vi "test_struct_abs_conventional.vi"() -> ()   [LabVIEW 2017]
doc: "Minimal example that demonstrates functions implemented in the SorpPropLib for absorption working pairs based on the conventional approach."
panel:
  out "Der. of concentration wrt. pressure":cluster{dbl[], dbl[]}[](graph)
  out "Der. of concentration wrt. temperature":cluster{dbl[], dbl[]}[](graph)
  out "Der. of pressure wrt. concentration":cluster{dbl[], dbl[]}[](graph)
  out "Der. of pressure wrt. temperature":cluster{dbl[], dbl[]}[](graph)
  out "Temperature":cluster{dbl[], dbl[]}[](graph)
  out "Pressure":cluster{dbl[], dbl[]}[](graph)
  out "Concentration":cluster{dbl[], dbl[]}[](graph)
  in  "WorkingPair (Input)":T1={"no_iso"=1, "no_p_sat"=1, "path_db"="D:\\Driesel\\SorpLibLocal\\labview_wrapper\\data\\json\\sorpproplib.json", "wp_as"="NaOH-KOH-CsOH", "wp_st"="", "wp_iso"="Duehring", "wp_rf"="Water", "rf_rhol"="SaturatedLiquidDensity_EoS1", "no_rhol"=1, "rf_psat"="VaporPressure_EoS1"}
  in  "Temperature in K (Input)":dbl=353.0
  in  "Pressure in Pa (Input)":dbl=1000.0
  # "Increase pressure by 5000 Pa in steps of 1 Pa."
  # "Path to database"
  # "Name of sorbent"
  # "Name of sub-type of sorbent"
  # "Name of refrigerant"
  # "Name of isotherm"
  # "ID of isotherm"
  # "Name of calculation approach for vapor pressure"
  # "ID of vapor pressure equation"
  # "Name of calculation approach for liquid density"
  # "ID of liquid density equation"
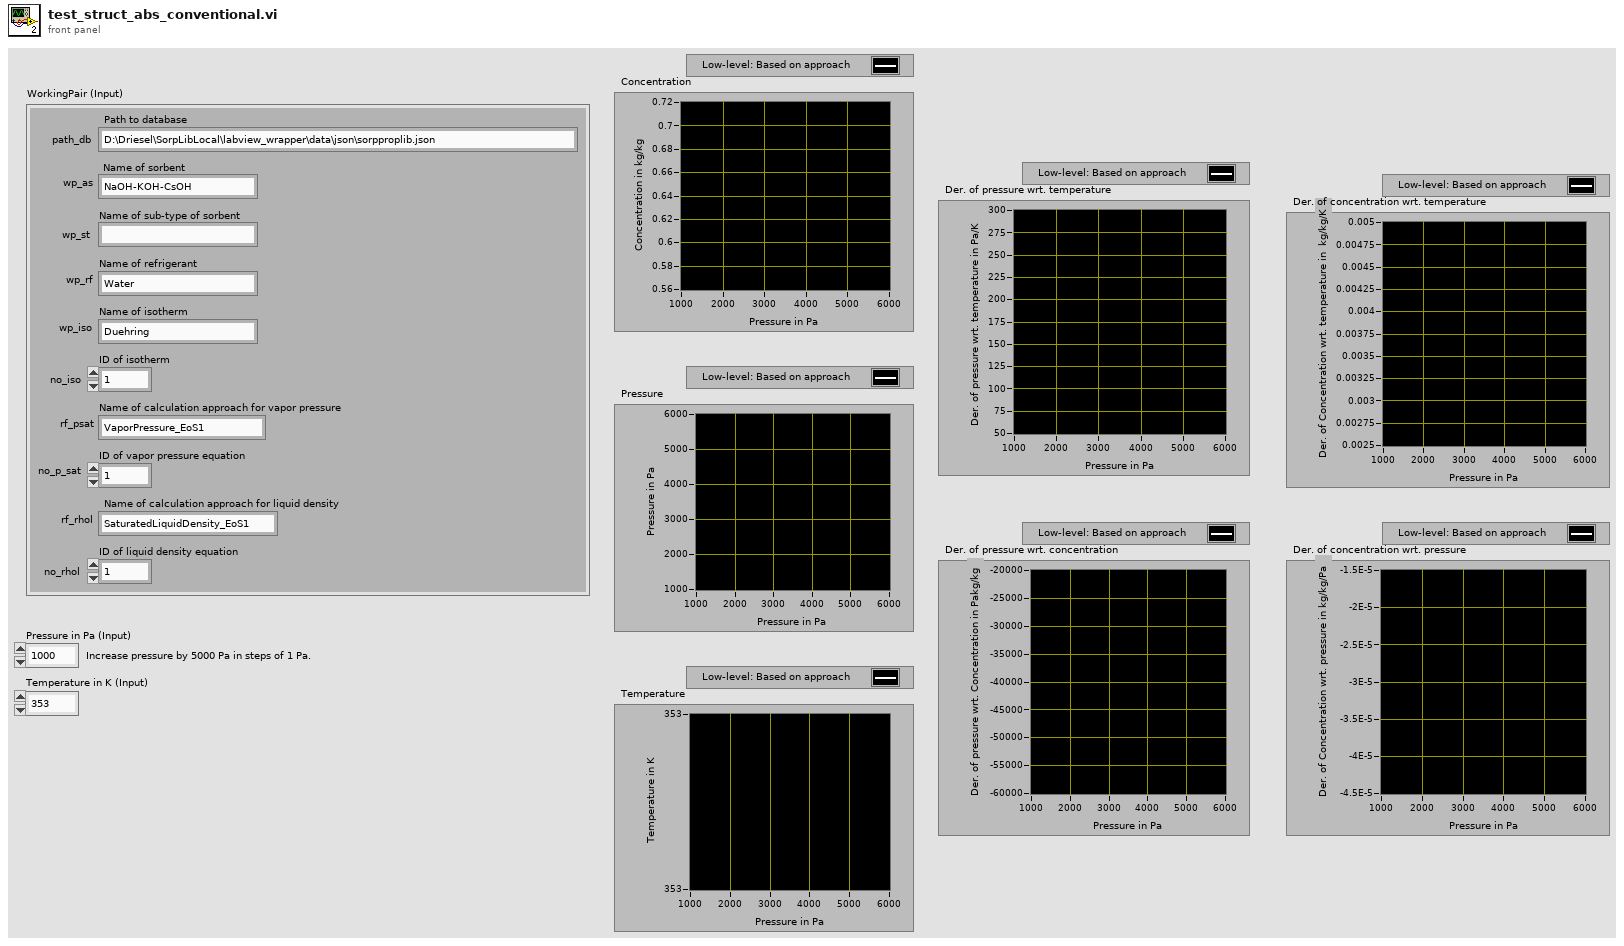
[diagram p1: front panel]
types:
  T1 = cluster{"no_iso":i32, "no_p_sat":i32, "path_db":string, "wp_as":string, "wp_st":string, "wp_iso":string, "wp_rf":string, "rf_rhol":string, "no_rhol":i32, "rf_psat":string}
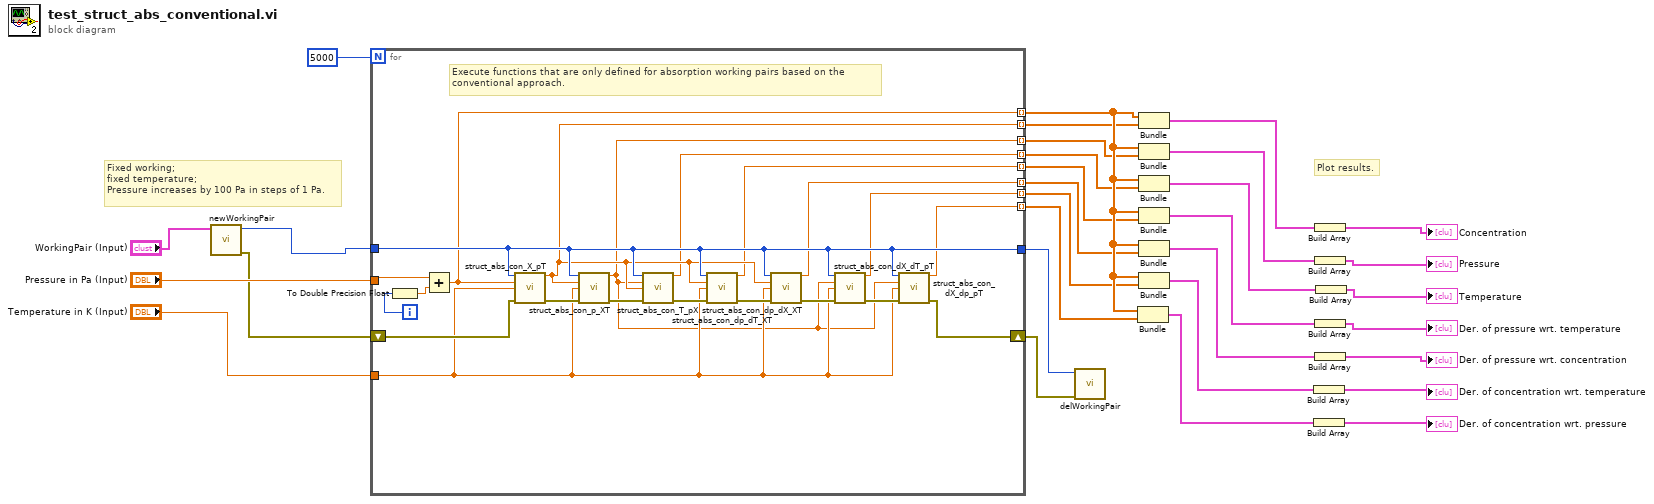
[diagram p0: block diagram]
diagram:
  # "Plot results."
  # "Fixed working;\nfixed temperature;\nPressure increases by 100 Pa in steps of 1 Pa."
  n1 = call "newWorkingPair.vi"("WorkingPair (Input)"="WorkingPair (Input)") -> ("Error (Output)"=w17:errorcluster, "workingPair"=w18:i64)  [unwired: 9 in]
  n2 = for {
    N: 5000 -> [_]
    tunnel: "Pressure in Pa (Input)" -> [w51]
    tunnel: "Temperature in K (Input)" -> [w38]
    tunnel: w18 -> [w40]
    shift-right: [w41] -> w16
    shift-left: w17 -> [w48]
    tunnel: [w39] -> w28 mode=indexing
    tunnel: [w40] -> w15
    tunnel: [w37] -> w14 mode=indexing
    tunnel: [w36] -> w13 mode=indexing
    tunnel: [w35] -> w12 mode=indexing
    tunnel: [w34] -> w11 mode=indexing
    tunnel: [w33] -> w10 mode=indexing
    tunnel: [w32] -> w9 mode=indexing
    tunnel: [w31] -> w8 mode=indexing
    i -> [w50]
    # "Execute functions that are only defined for absorption working pairs based on the\nconventional approach."
    n3 = To Double Precision Float(number=w50) -> (double precision float=w49:dbl)
    n4 = Add(x=w51, y=w49) -> (x+y=w39:dbl)
    n5 = call "struct_abs_con_X_pT.vi"("Reference working pair (Input)"=w40, "Pressure in Pa (Input)"=w39, "Temperature in K (Input)"=w38, "Error (Input)"=w48) -> ("Concentration in kg/kg (Output)"=w37:dbl, "Error (Output)"=w47:errorcluster)  [unwired: 10 in]
    n6 = call "struct_abs_con_p_XT.vi"("Reference working pair (Input)"=w40, "Concentration in kg/kg (Input)"=w37, "Temperature in K (Input)"=w38, "Error (Input)"=w47) -> ("Pressure in Pa (Output)"=w36:dbl, "Error (Output)"=w46:errorcluster)  [unwired: 10 in]
    n7 = call "struct_abs_con_T_pX.vi"("Reference working pair (Input)"=w40, "Pressure in Pa (Input)"=w36, "Concentration in kg/kg (Input)"=w37, "Error (Input)"=w46) -> ("Temperature in K (Output)"=w35:dbl, "Error (Output)"=w45:errorcluster)  [unwired: 10 in]
    n8 = call "struct_abs_con_dp_dT_XT.vi"("Reference working pair (Input)"=w40, "Concentration in kg/kg (Input)"=w37, "Temperature in K (Input)"=w38, "Error (Input)"=w45) -> ("Der. of equilibrium pressure wrt. temperature in Pa/K (Output)"=w34:dbl, "Error (Output)"=w44:errorcluster)  [unwired: 10 in]
    n9 = call "struct_abs_con_dp_dX_XT.vi"("Reference working pair (Input)"=w40, "Concentration in kg/kg (Input)"=w37, "Temperature in K (Input)"=w38, "Error (Input)"=w44) -> ("Der. of equilibrium pressure wrt. concentration in Pakg/kg (Output)"=w33:dbl, "Error (Output)"=w43:errorcluster)  [unwired: 10 in]
    n10 = call "struct_abs_con_dX_dT_pT.vi"("Reference working pair (Input)"=w40, "Pressure in Pa (Input)"=w36, "Temperature in K (Input)"=w38, "Error (Input)"=w43) -> ("Der. of equilibrium concentration wrt. temperature in kg/kg/K (Output)"=w32:dbl, "Error (Output)"=w42:errorcluster)  [unwired: 10 in]
    n11 = call "struct_abs_con_dX_dp_pT.vi"("Reference working pair (Input)"=w40, "Pressure in Pa (Input)"=w36, "Temperature in K (Input)"=w38, "Error (Input)"=w42) -> ("Der. of equilibrium concentration wrt. pressure in kg/kg/Pa (Output)"=w31:dbl, "Error (Output)"=w41:errorcluster)  [unwired: 10 in]
  }
  n12 = call "delWorkingPair.vi"("Error (Input)"=w16, "workingPair"=w15) -> ()  [unwired: 9 in, 1 out]
  n13 = Bundle(w28, w8) -> (w21:cluster{dbl[], dbl[]})  [unwired: 1 in]
  n14 = Bundle(w28, w14) -> (w27:cluster{dbl[], dbl[]})  [unwired: 1 in]
  n15 = Bundle(w28, w13) -> (w26:cluster{dbl[], dbl[]})  [unwired: 1 in]
  n16 = Bundle(w28, w12) -> (w25:cluster{dbl[], dbl[]})  [unwired: 1 in]
  n17 = Bundle(w28, w11) -> (w24:cluster{dbl[], dbl[]})  [unwired: 1 in]
  n18 = Bundle(w28, w10) -> (w23:cluster{dbl[], dbl[]})  [unwired: 1 in]
  n19 = Bundle(w28, w9) -> (w22:cluster{dbl[], dbl[]})  [unwired: 1 in]
  n20 = Build Array(w22) -> (→"Der. of concentration wrt. temperature":cluster{dbl[], dbl[]}[])
  n21 = Build Array(w21) -> (→"Der. of concentration wrt. pressure":cluster{dbl[], dbl[]}[])
  n22 = Build Array(w27) -> (→"Concentration":cluster{dbl[], dbl[]}[])
  n23 = Build Array(w26) -> (→"Pressure":cluster{dbl[], dbl[]}[])
  n24 = Build Array(w24) -> (→"Der. of pressure wrt. temperature":cluster{dbl[], dbl[]}[])
  n25 = Build Array(w23) -> (→"Der. of pressure wrt. concentration":cluster{dbl[], dbl[]}[])
  n26 = Build Array(w25) -> (→"Temperature":cluster{dbl[], dbl[]}[])
